vi "Density meter func glob.vi"(2 "Sample DateTime in":timestamp, 3 "Density in":dbl, 4 "Action":enum16{"Get", "Set"}(ring)) -> (0 "Sample DateTime out":timestamp, 1 "Density out":dbl)   [LabVIEW 2011]
panel:
  # "by Paul Nathan, 06/03/2012"
  # "Revisions:\nDate       Desc.      Auth.\nx               x               x"
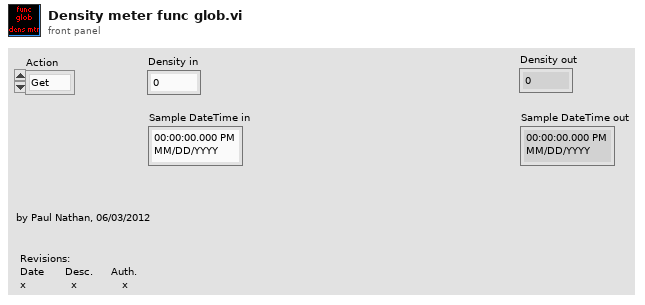
[diagram p1: front panel]
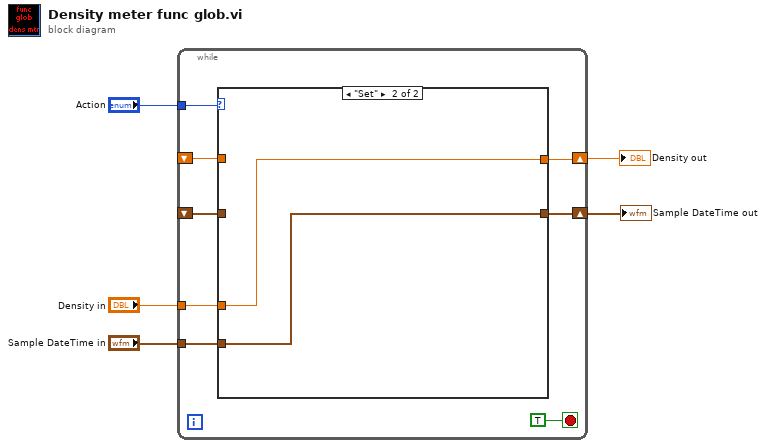
[diagram p0: block diagram]
diagram:
  n1 = while {
    tunnel: "Action" -> [w12]
    shift-right: [w11] -> w3
    shift-left: _ -> [w10]
    tunnel: "Density in" -> [w9]
    shift-right: [w7] -> w1
    shift-left: _ -> [w8]
    tunnel: "Sample DateTime in" -> [w6]
    stop <- TRUE stop-if-true
    n2 = case shown="\"Set\"" w12 {
      tunnel: [w15 w17] -> w11
      tunnel: w10 -> [w15 _]
      tunnel: w9 -> [_ w17]
      tunnel: w8 -> [w14 _]
      tunnel: [w14 w16] -> w7
      tunnel: w6 -> [_ w16]
      frame "Get" {
      }
      frame "Set" {
      }
    }
  }
  "Density out" <- w3
  "Sample DateTime out" <- w1
